vi "List Tester - Subpanel.vi"() -> ()   [LabVIEW 2016]
uses:
  HorizontalList.xctl
panel:
  in  "HorizontalList":i32(xcontrol)
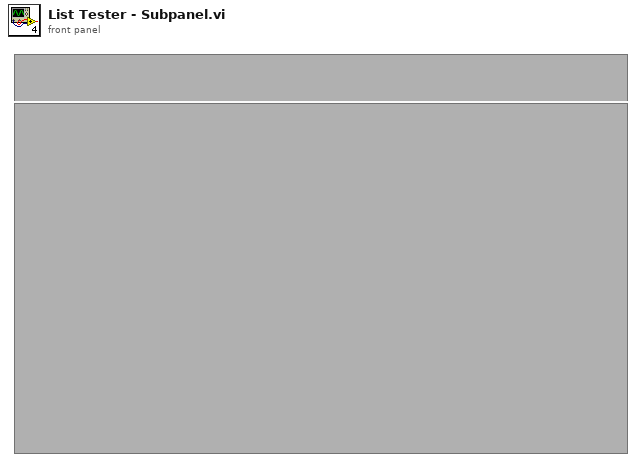
[diagram p1: front panel]
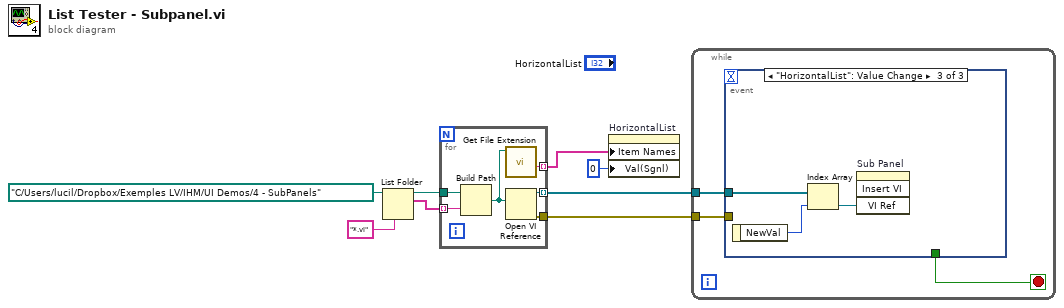
[diagram p0: block diagram]
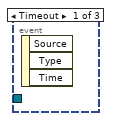
[diagram p2: hidden frame]
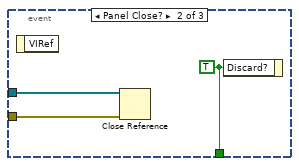
[diagram p3: hidden frame]
diagram:
  n1 = List Folder(path=path "C:/Users/lucil/Dropbox/Exemples LV/IHM/UI Demos/4 - SubPanels", pattern="*.vi") -> (path out=w7:path, filenames=w6:string[])  [unwired: 2 in, 2 out]
  n2 = for {
    tunnel: w7 -> [w14]
    tunnel: w6 -> [w13] mode=indexing
    tunnel: [w11] -> w5 mode=indexing
    tunnel: [w10] -> w3 mode=indexing
    tunnel: [w9] -> w1
    n3 = Build Path(base path=w14, name or relative path=w13) -> (appended path=w12:path)
    n4 = call <vilib>:"Get File Extension.vi"("file"=w12) -> ("filename without extension"=w11:string)  [unwired: 6 in, 4 out]
    n5 = Open VI Reference(vi path=w12) -> (vi reference=w10:refnum<vi>, error out=w9:errorcluster)  [unwired: 5 in]
  }
  n6 = property on="HorizontalList" class="HorizontalList (strict)"("Item Names"=w5, "Val(Sgnl)"=0 ("Value (Signaling)")) -> ()  [unwired: 2 in, 2 out]
  n7 = while {
    tunnel: w3 -> [w16]
    tunnel: w1 -> [w15]
    stop <- w17 stop-if-true
    n8 = event shown="[2] \"HorizontalList\": Value Change" {
      selector: _ -> [_ _ _]
      dyn-events: _ -> [_ _ _]
      timeout: _ -> [_ _ _]
      tunnel: [_ w20 _] -> w17
      tunnel: w16 -> [_ w19 w23]
      tunnel: w15 -> [_ w18 _]
      event Timeout {
        n9 = event-data() -> ()  [unwired: 1 in, 3 out]
      }
      event Panel Close? {
        w20 = TRUE ("Discard?")
        n10 = event-data() -> ()  [unwired: 1 in, 1 out]
        n11 = Close Reference(reference=w19, error in (no error)=w18) -> ()  [unwired: 1 out]
        n12 = event-data("Discard?"=w20) -> ()  [unwired: 1 in, 1 out]
      }
      event "HorizontalList": Value Change {
        n13 = event-data() -> ("NewVal"=w22:i32)  [unwired: 1 in]
        n14 = Index Array(array=w23, index=w22) -> (element=w21:refnum<vi>)
        n15 = invoke on="Sub Panel" class="SubPnl" method="Insert VI"("VI Ref"=w21) -> ()  [unwired: 3 in, 4 out]
      }
    }
  }
